vi "Pre Launch Init.vi"(11 "client in":refnum<class "client.lvclass">) -> (0 "error out":errorcluster, 3 "client out":refnum<class "client.lvclass">)   [LabVIEW 2016, in "client.lvlib" / "client.lvclass"]
doc: "(<B>Filename</B>: Actor Framework.lvlib:Actor.lvclass:Pre Launch Init.vi)\n\nDefines behavior that occurs after the Launch Nested Actor method is invoked but before the actor's Actor Core method begins running.\n\nBy default, this method does nothing. A descendant class may override it to define behavior."
uses:
  client.lvclass
  client.lvclass/client.ctl
  <vilib>/ActorFramework/Actor/Actor.lvclass
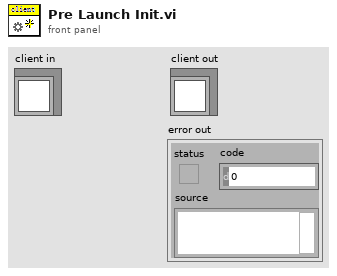
[diagram p1: front panel]
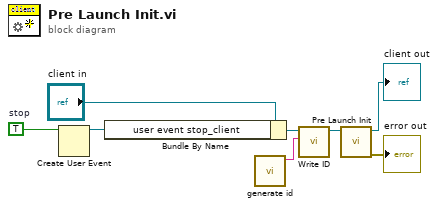
[diagram p0: block diagram]
diagram:
  w6 = TRUE  # stop
  n1 = Create User Event(user event datatype=w6) -> (user event=w5:refnum<user-event>)  [unwired: 1 in, 1 out]
  n2 = Bundle By Name(cluster="client in", "user event stop_client"=w5) -> (w3:refnum<class "client.lvclass">)
  n3 = call "generate id.vi"() -> ("id"=w1:string)  [unwired: 11 in]
  n4 = call-dynamic "Write ID.vi"("ID"=w1, "client in"=w3) -> ("client out"=w2:refnum<class "client.lvclass">)  [unwired: 8 in, 1 out]
  n5 = call-parent "Pre Launch Init.vi"("Actor in"=w2) -> ("error out"=→"error out":errorcluster, "Actor out"=→"client out":refnum<class "client.lvclass">)  [unwired: 9 in]
